vi "calibration.vi"(0 "信号时长[s]":dbl, 1 "Buffer":T1={"# buffers"=4, "Buffer size"=2048, "unit (ms)"=enum."Samples"}, 5 "终止频率[Hz]":dbl, 9 "起始频率[Hz]":dbl, 11 "信号幅值[V]":dbl, 13 "format":cluster{"Rate":i32, "Bits":i32, "Channels":u32}) -> ()   [LabVIEW 2021]
uses:
  Global.vi
  <vilib>/addons/_NISVFA/_Generation/SoundVib_Generation.lvlib
  <vilib>/Analysis/NI_AALPro.lvlib
  <vilib>/measure/NI_MABase.lvlib
panel:
  in  "Close Square":bool
  in  "校准电压值":dbl[](array[numeric])
  in  "amp":dbl
  in  "开始校准":bool
  in  "Stop":bool
  in  "验证校准值":bool
  out "Calibration Curve":cluster{"X":dbl, "Y":dbl}[](graph)
  out "intercept":dbl
  out "slope":dbl
  out "校准中":string
  # "-step1:  将万用表调整到交流电压测试模式，将信号输出连接万用表；\n-step2：点击开始校准按钮，待万用表示数稳定，点击暂停按钮，记录最大测量电压值；\n-step3：将校准电压值填入弹出的对话框；\n-step4：重复step2-step3 3次，校准结束后软件自动计算校准曲线；\n-step5：点击验证校准值，查看万用表示数是否与信号幅值相同；\n-step6：点击暂停并选择是否保存校准曲线"
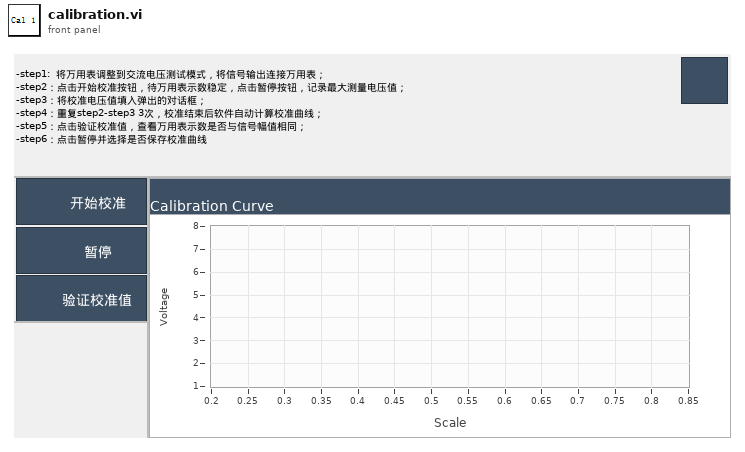
[diagram p1: front panel]
types:
  T1 = cluster{"# buffers":i32, "Buffer size":i32, "unit (ms)":enum16{"time (ms)", "Samples"}}
  T2 = cluster{"slope":dbl, "intercept":dbl, "校准电压值":dbl[]}
  T3 = typedef "SoundHandle.ctl" = cluster{"DeviceID":u16, "Samples/buf":u32, "Sampl rate":u32, "Bits/sample":u16, "Channels":u8, "Opened":bool}
  T4 = cluster{"start frequency [Hz]":dbl, "stop frequency [Hz]":dbl}
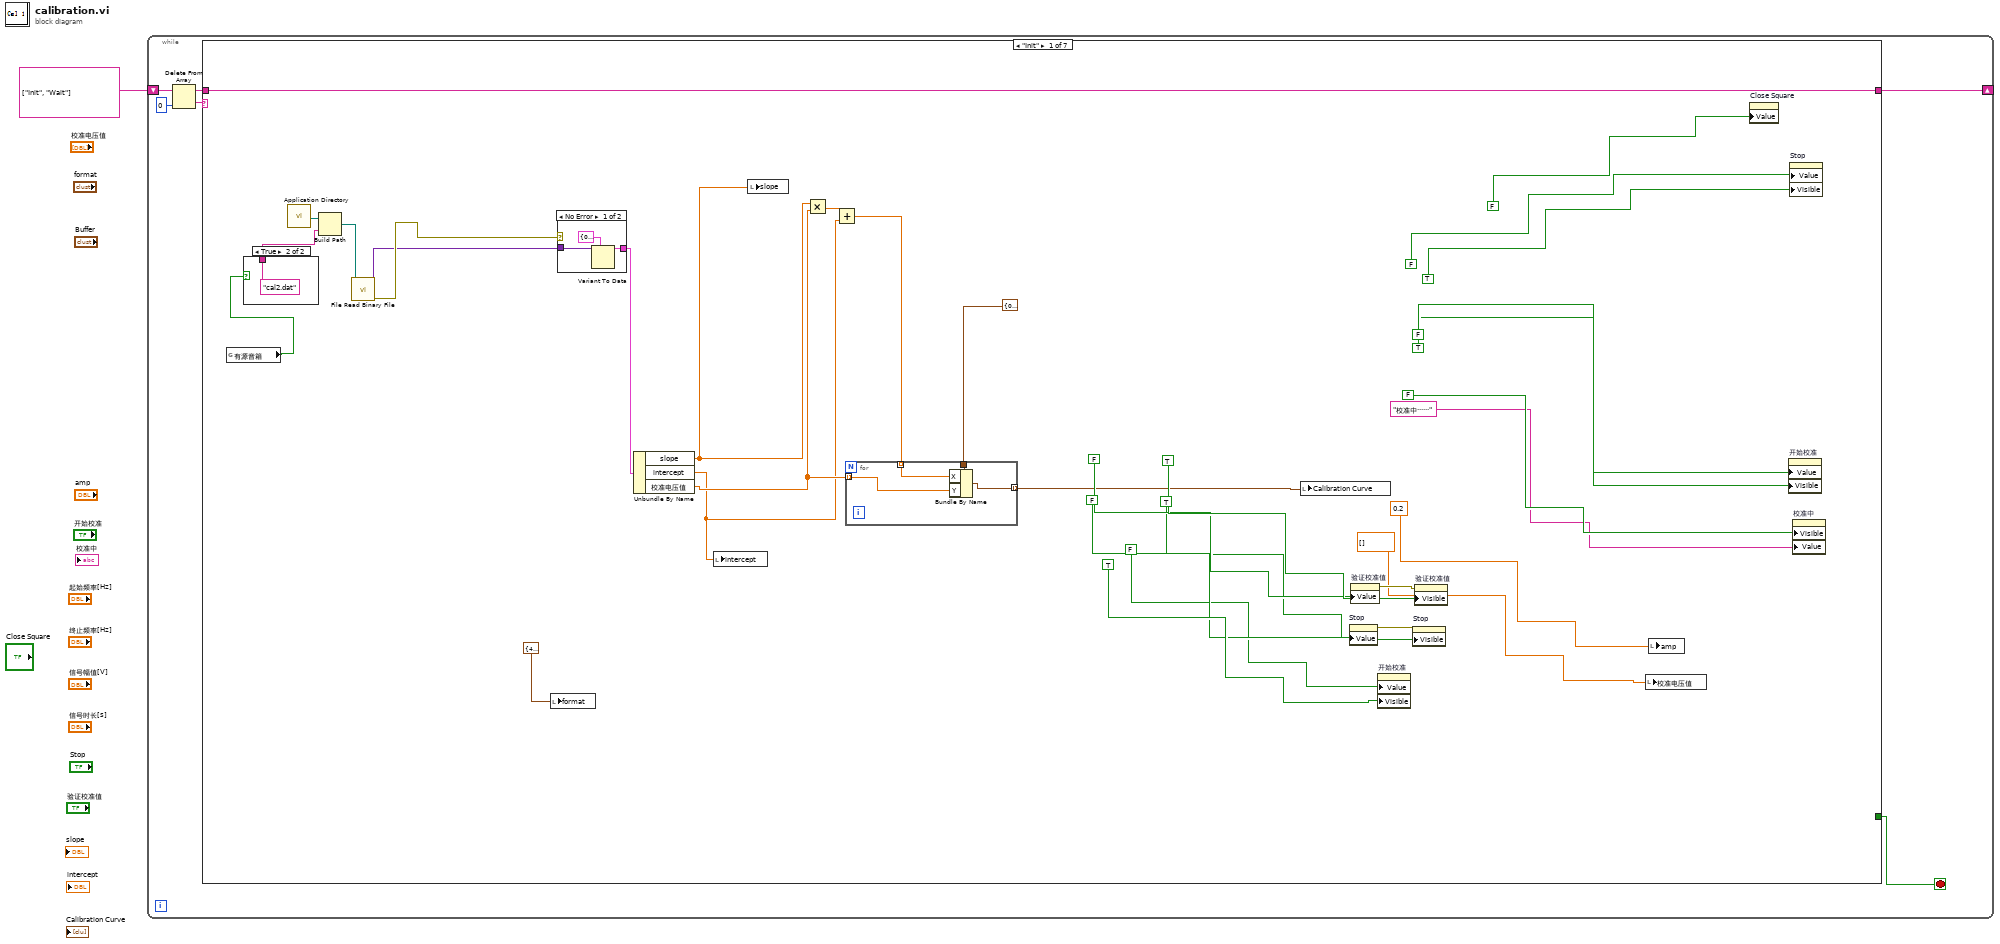
[diagram p0: block diagram]
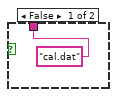
[diagram p2: hidden frame]
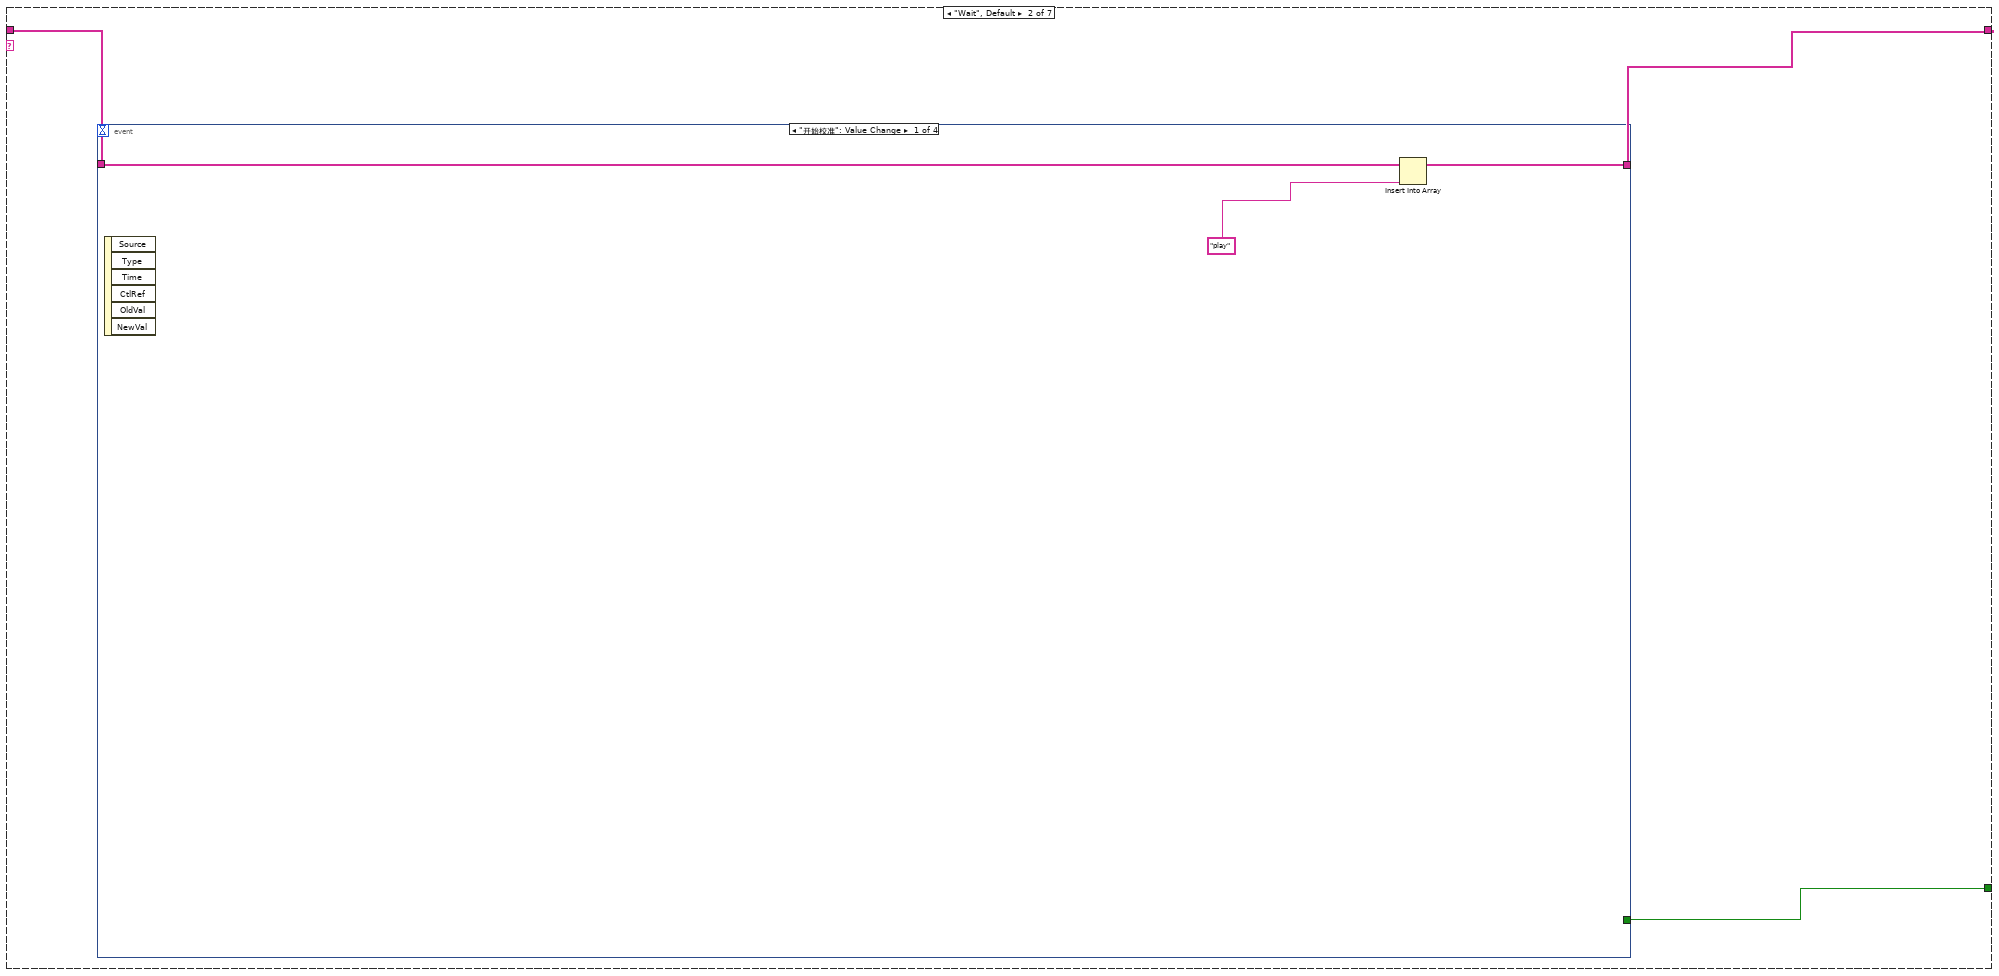
[diagram p4: hidden frame]
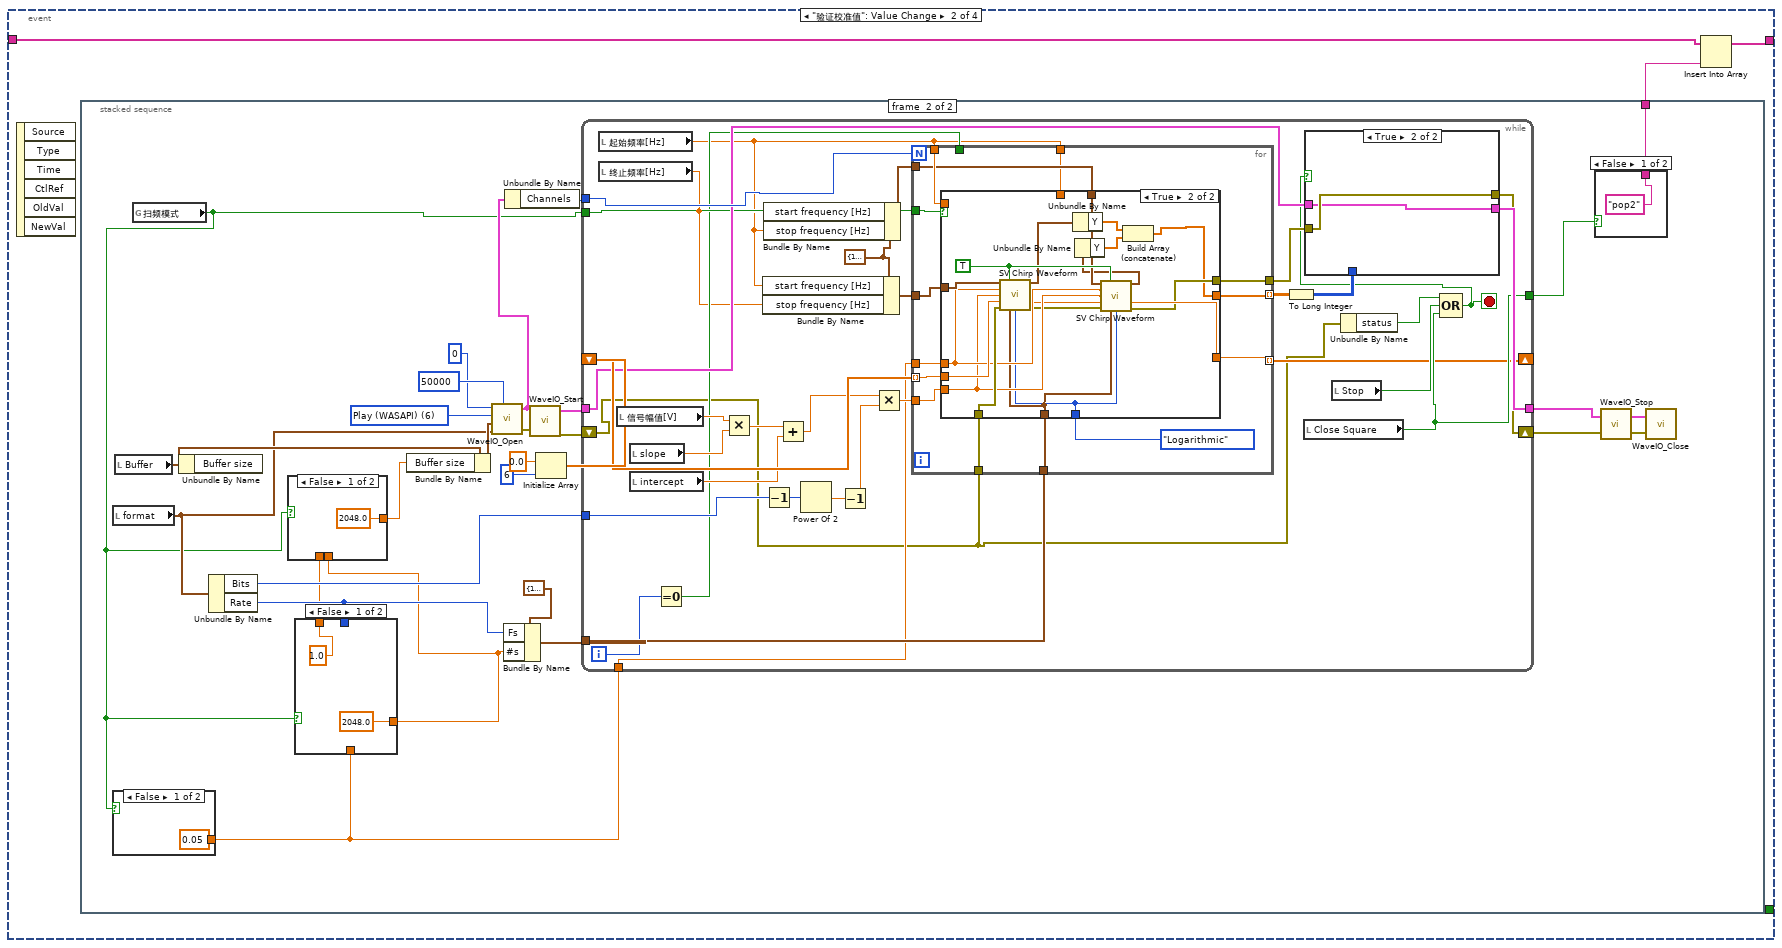
[diagram p5: hidden frame]
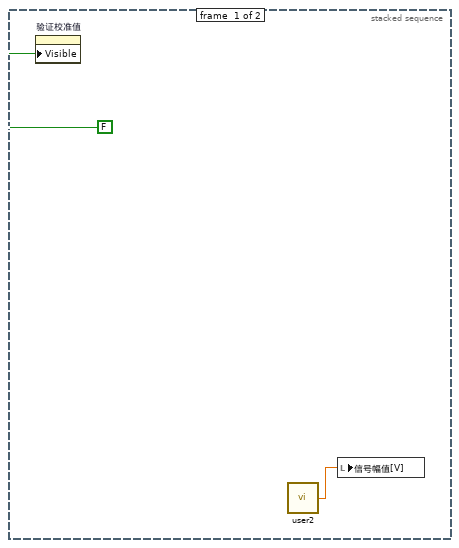
[diagram p6: hidden frame]
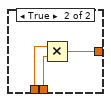
[diagram p7: hidden frame]
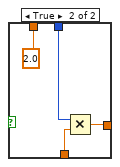
[diagram p8: hidden frame]
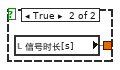
[diagram p9: hidden frame]
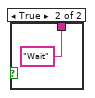
[diagram p10: hidden frame]
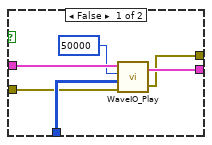
[diagram p11: hidden frame]
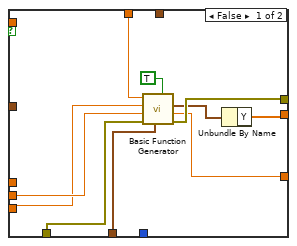
[diagram p12: hidden frame]
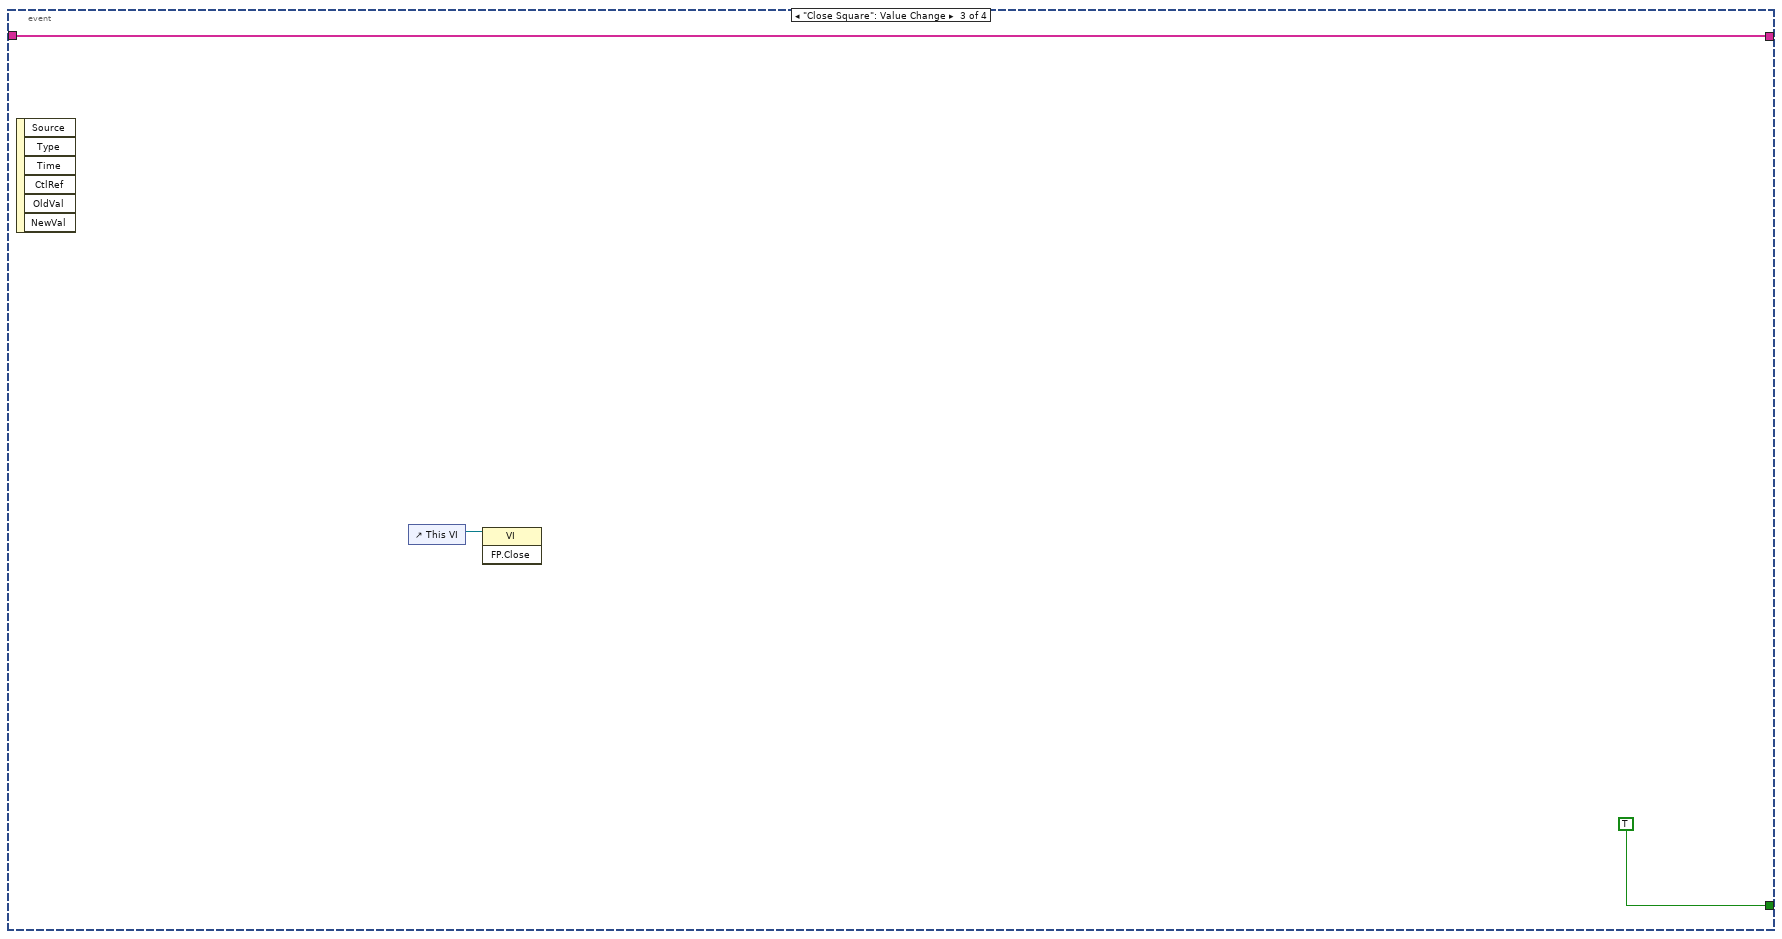
[diagram p13: hidden frame]
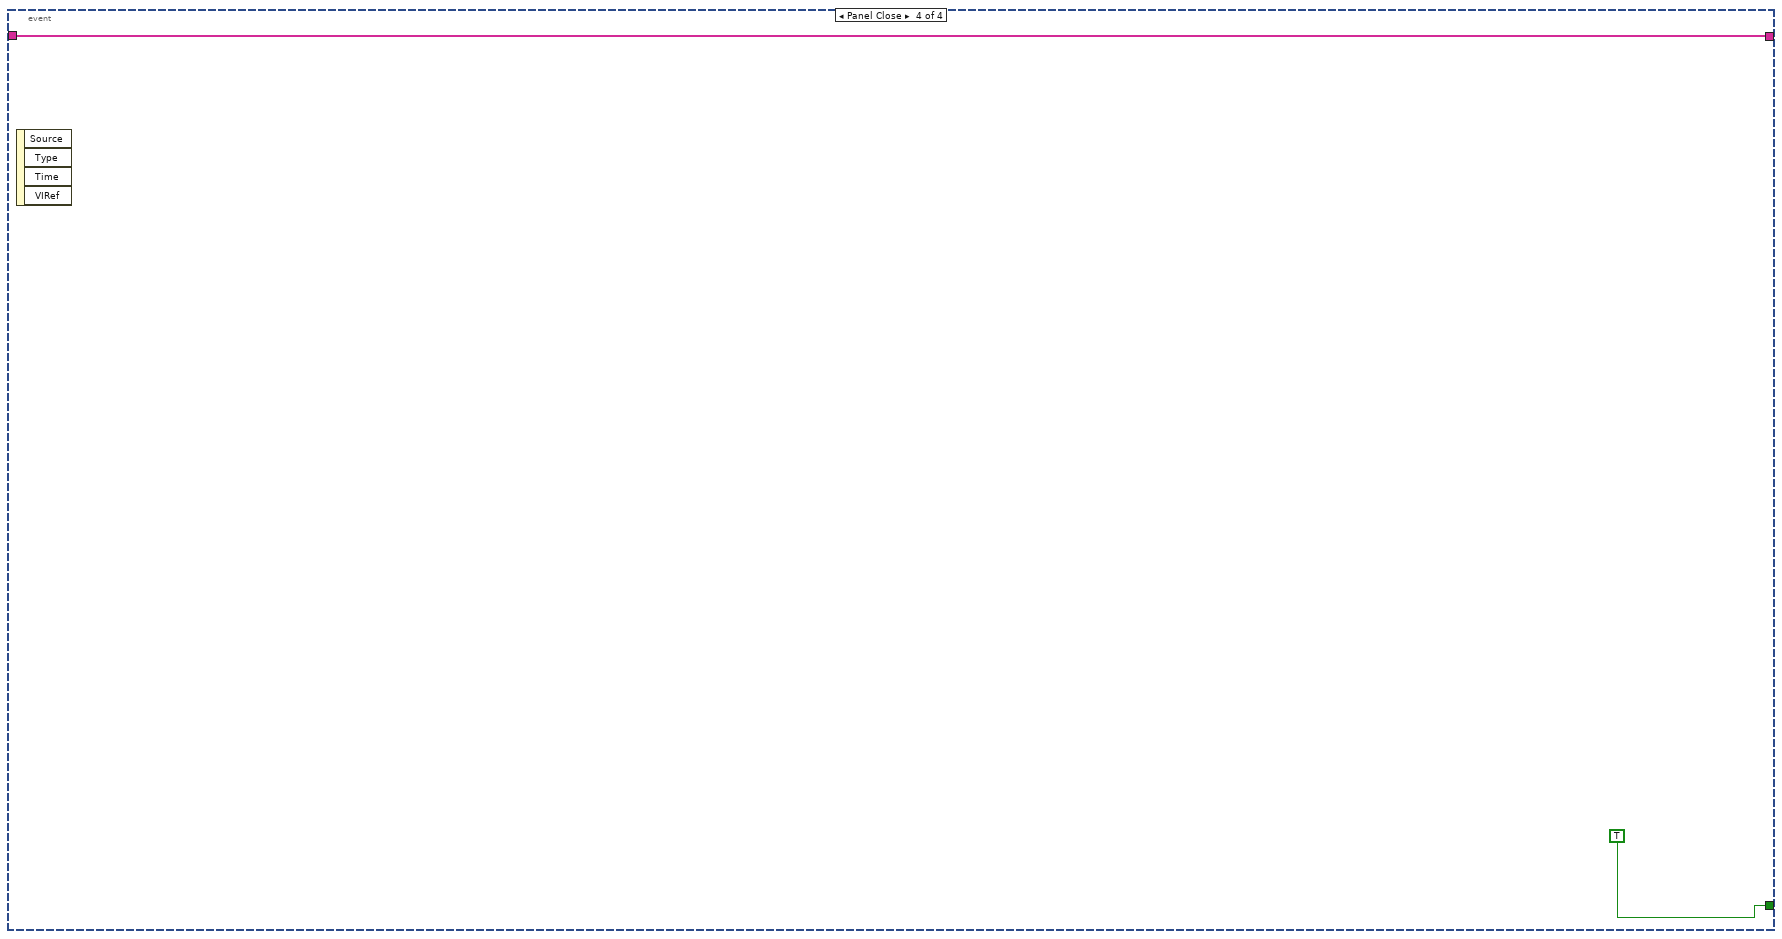
[diagram p14: hidden frame]
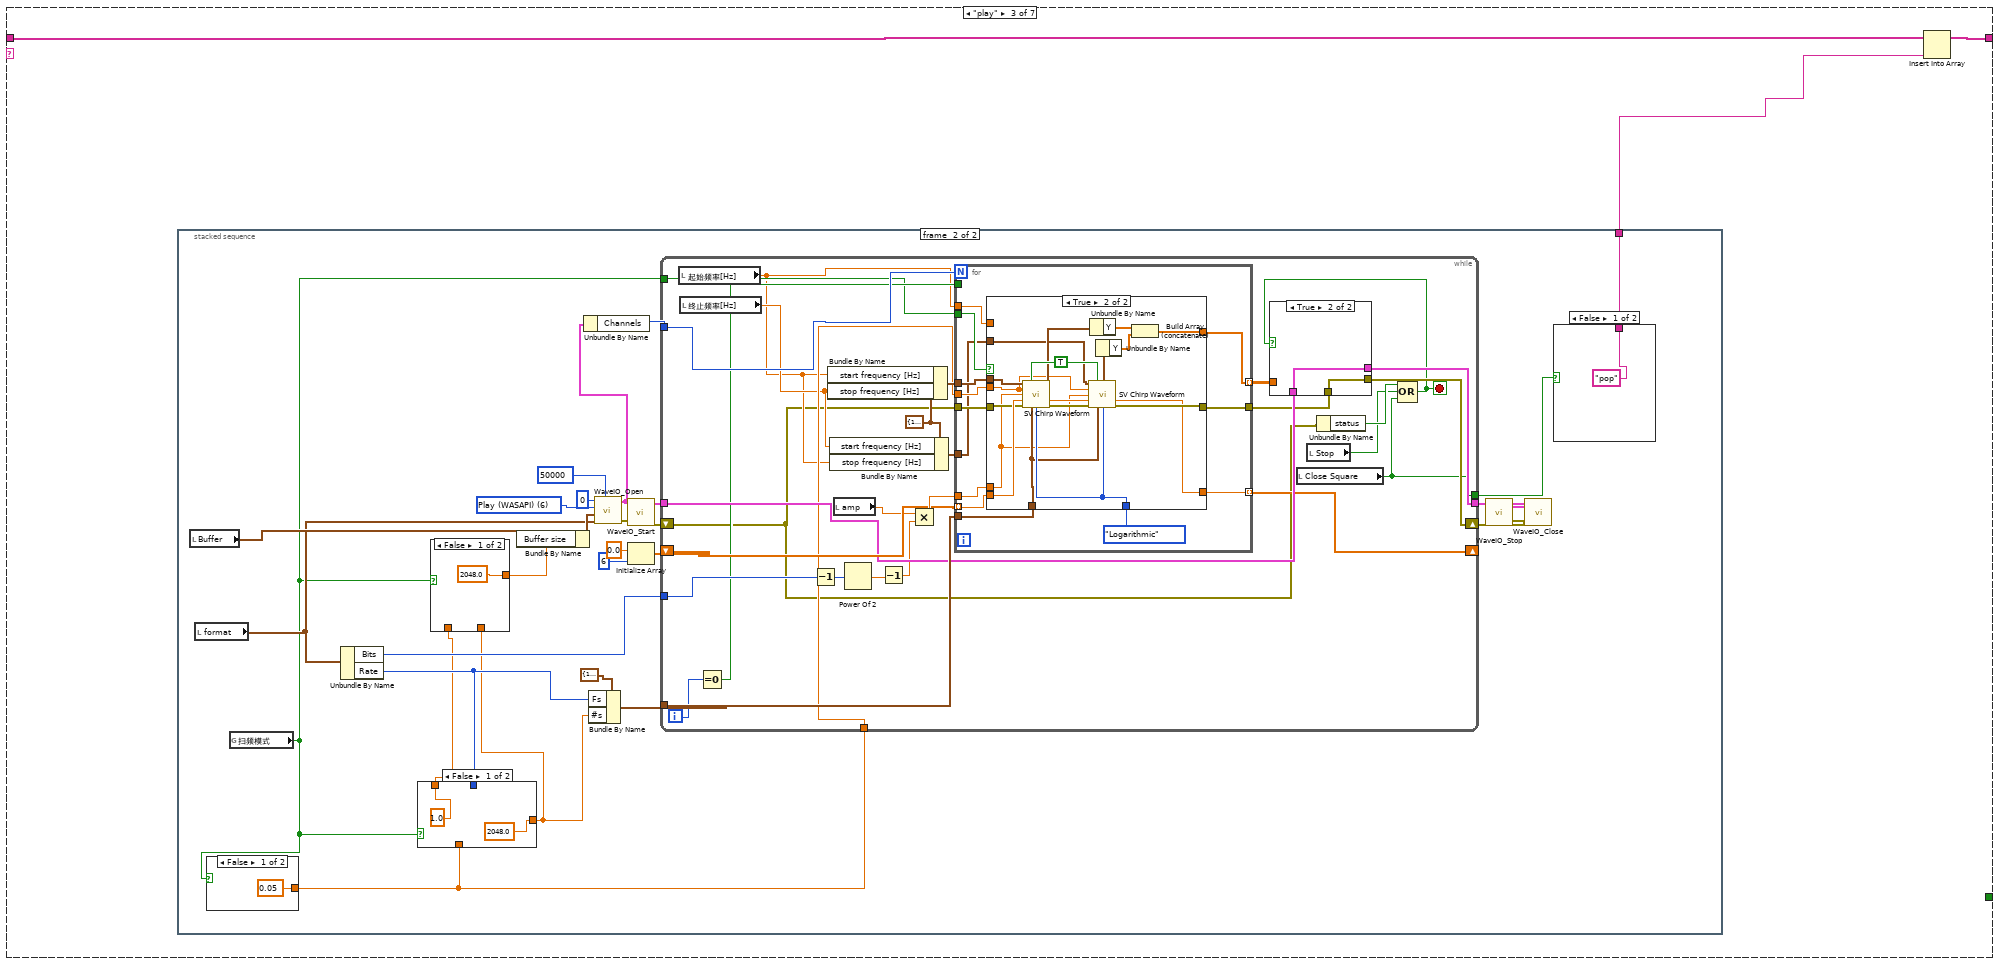
[diagram p15: hidden frame]
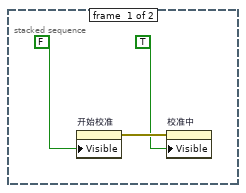
[diagram p16: hidden frame]
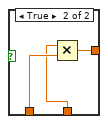
[diagram p17: hidden frame]
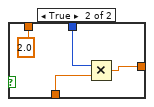
[diagram p18: hidden frame]
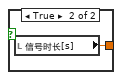
[diagram p19: hidden frame]
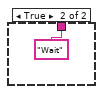
[diagram p20: hidden frame]
diagram:
  n1 = while {
    shift-right: [w3] -> _
    shift-left: string[] ["Init", "Wait"] -> [w6]
    stop <- w2 stop-if-true
    n2 = Delete From Array(array=w6, index=0 ("索引")) -> (deleted portion=w5:string, array with subset deleted=w4:string[])  [unwired: 1 in]
    n3 = case shown="\"Init\"" w5 {
      tunnel: [_ w50 _ TRUE _ _ _] -> w2
      tunnel: w4 -> [w31 w52 w195 w320 w328 w345 w386]
      tunnel: [w31 w51 w194 w320 w326 w344 w386] -> w3
      frame "Init" {
        n4 = global read "Global.vi" "有源音箱"() -> (w8:bool)
        n5 = case shown="True" w8 {
          tunnel: ["cal.dat" ("名称或相对路径") "cal2.dat" ("名称或相对路径")] -> w23
          frame False {
          }
          frame True {
          }
        }
        n6 = call <vilib>:"Application Directory.vi"() -> ("Application Directory"=w24:path)
        n7 = Build Path(base path=w24, name or relative path=w23) -> (appended path=w25:path)
        n8 = call "File Read Binary File.vi"("file path"=w25) -> ("error Output"=w28:errorcluster, "Variant Output"=w26:variant)  [unwired: 8 in, 1 out]
        n9 = local write "format"(cluster{"Rate":i32, "Bits":i32, "Channels":u32} {"Rate"=44100, "Bits"=24, "Channels"=2} ("format")) -> ()
        n10 = case shown="No Error" w28 {
          tunnel: w26 -> [w49 _]
          tunnel: [w48 _] -> w27
          frame No Error {
            n11 = Variant To Data(type=T2 {"slope"=0.0, "intercept"=0.0, "校准电压值"=[3.37, 6.73, 10.1, 13.48]}, Variant=w49) -> (data=w48:T2)  [unwired: 1 in, 1 out]
          }
          frame Error {
          }
        }
        n12 = Unbundle By Name(w27) -> ("slope"=w17:dbl, "intercept"=w16:dbl, "校准电压值"=w18:dbl[])
        n13 = local write "intercept"(w16) -> ()
        n14 = local write "slope"(w17) -> ()
        n15 = Multiply(x=w17, y=w18) -> (x*y=w22:dbl[])
        n16 = Add(x=w22, y=w16) -> (x+y=w21:dbl[])
        n17 = for {
          tunnel: cluster{"X":dbl, "Y":dbl} {"X"=0.0, "Y"=0.0} -> [w46]
          tunnel: w18 -> [w43] mode=indexing
          tunnel: w21 -> [w44] mode=indexing
          tunnel: [w45] -> w20 mode=indexing
          n18 = Bundle By Name(cluster=w46, "X"=w44, "Y"=w43) -> (w45:cluster{"X":dbl, "Y":dbl})
        }
        n19 = local write "Calibration Curve"(w20) -> ()
        n20 = property on="Stop" class="Bool (strict)"("Value"=FALSE ("可见")) -> (error out=w11:errorcluster)  [unwired: 2 in, 1 out]
        n21 = property on="验证校准值" class="Bool (strict)"("Value"=FALSE ("可见")) -> (error out=w40:errorcluster)  [unwired: 2 in, 1 out]
        n22 = property on="开始校准" class="Bool (strict)"("Value"=FALSE ("开始校准"), "Visible"=TRUE) -> ()  [unwired: 2 in, 2 out]
        n23 = property on="Stop" class="Bool (strict)"(error in=w11, "Visible"=TRUE) -> ()  [unwired: 1 in, 2 out]
        n24 = property on="验证校准值" class="Bool (strict)"(error in=w40, "Visible"=TRUE) -> ()  [unwired: 1 in, 2 out]
        n25 = local write "校准电压值"(dbl[] [] ("Array")) -> ()
        n26 = local write "amp"(0.2 ("amp")) -> ()
        n27 = property on="Close Square" class="Bool (strict)"("Value"=FALSE ("Close Square")) -> ()  [unwired: 2 in, 2 out]
        n28 = property on="开始校准" class="Bool (strict)"("Value"=FALSE, "Visible"=TRUE ("可见")) -> ()  [unwired: 2 in, 2 out]
        n29 = property on="Stop" class="Bool (strict)"("Value"=FALSE ("Stop"), "Visible"=TRUE) -> ()  [unwired: 2 in, 2 out]
        n30 = property on="校准中" class="Str"("Visible"=FALSE ("可见"), "Value"="校准中······" ("校准中")) -> ()  [unwired: 2 in, 2 out]
      }
      frame "Wait", Default {
        n31 = event shown="[0] \"开始校准\": Value Change" {
          selector: _ -> [_ _ _ _]
          dyn-events: _ -> [_ _ _ _]
          timeout: _ -> [_ _ _ _]
          tunnel: [_ _ TRUE TRUE] -> w50
          tunnel: [w54 w56 w188 w191] -> w51
          tunnel: w52 -> [w55 w58 w188 w191]
          event "开始校准": Value Change {
            n32 = event-data() -> ()  [unwired: 1 in, 6 out]
            n33 = Insert Into Array(array=w55, new element="play" ("new element/subarray")) -> (w54:string[])  [unwired: 1 in]
          }
          event "验证校准值": Value Change {
            n34 = event-data() -> ()  [unwired: 1 in, 6 out]
            n35 = stacked-sequence {
              tunnel: [_ w66] -> w57
              frame #0 {
                n36 = property on="验证校准值" class="Bool (strict)"("Visible"=FALSE ("可见")) -> ()  [unwired: 2 in, 2 out]
                n37 = call "user2.vi"() -> ("Numeric"=w59:dbl)
                n38 = local write "信号幅值[V]"(w59) -> ()
              }
              frame #1 {
                w72 = u16 6 items=["Record", "Play", "Loopback", "ASIO input", "ASIO output", "Record (WASAPI)", "Play (WASAPI)", "Record Combi", "Play Combi"] ("device type (Record)")
                n39 = local read "format"() -> (w68:cluster{"Rate":i32, "Bits":i32, "Channels":u32})
                n40 = local read "Buffer"() -> (w69:T1)
                n41 = global read "Global.vi" "扫频模式"() -> (w61:bool)
                n42 = case shown="False" w61 {
                  tunnel: [0.05 ("信号时长[s]") w101] -> w64
                  frame False {
                  }
                  frame True {
                    n43 = local read "信号时长[s]"() -> (w101:dbl)
                  }
                }
                n44 = Unbundle By Name(w69) -> ()  [unwired: 1 out]
                n45 = Unbundle By Name(w68) -> ("Bits"=w80:i32, "Rate"=w65:i32)
                n46 = case shown="False" w61 {
                  tunnel: [2048.0 w99] -> w63
                  tunnel: w65 -> [_ w98]
                  tunnel: w64 -> [_ w97]
                  tunnel: [1.0 ("x") 2.0 ("x")] -> w62
                  frame False {
                  }
                  frame True {
                    n47 = Multiply(x=w98, y=w97) -> (x*y=w99:dbl)
                  }
                }
                n48 = case shown="False" w61 {
                  tunnel: [2048.0 w93] -> w70
                  tunnel: w63 -> [_ w92]
                  tunnel: w62 -> [_ w91]
                  frame False {
                  }
                  frame True {
                    n49 = Multiply(x=w91, y=w92) -> (x*y=w93:dbl)
                  }
                }
                n50 = Bundle By Name(cluster=w69, "Buffer size"=w70) -> (w71:T1)
                n51 = call "WaveIO_Open.vi"("idev"=u32 0, "Watchdog timeout (msec) (default=OFF)"=50000, "device type (Record)"=w72, "Buffer Config"=w71, "Format (44kHz, 16Bit, stereo)"=w68) -> ("Sound Handle Out"=w75:T3, "error out"=w82:errorcluster)  [unwired: 2 in]
                n52 = Bundle By Name(cluster=cluster{"Fs":dbl, "#s":dbl} {"Fs"=1000.0, "#s"=1000.0} ("sampling info"), "Fs"=w65, "#s"=w63) -> (w85:cluster{"Fs":dbl, "#s":dbl})
                n53 = Unbundle By Name(w75) -> ("Channels"=w74:u8)
                n54 = call "WaveIO_Start.vi"("error in (no error)"=w82, "Handle"=w75) -> ("error out"=w83:errorcluster, "Handle Out"=w84:T3)
                n55 = Initialize Array(0.0 ("element"), 6 ("dimension size")) -> (w79:dbl[])
                n56 = while {
                  shift-right: [w129] -> w81
                  shift-left: w83 -> [w105]
                  tunnel: w84 -> [w127]
                  tunnel: [w136] -> w88
                  tunnel: w85 -> [w137]
                  tunnel: w80 -> [w135]
                  shift-right: [w107] -> _
                  shift-left: w79 -> [w130]
                  tunnel: w74 -> [w128]
                  tunnel: w64 -> [w123]
                  tunnel: [w115] -> w67
                  tunnel: w61 -> [w113]
                  i -> [w112]
                  stop <- w104 stop-if-true
                  w110 = T4 {"start frequency [Hz]"=10.0, "stop frequency [Hz]"=10000.0} ("frequency range")
                  n57 = local read "起始频率[Hz]"() -> (w106:dbl)
                  n58 = local read "终止频率[Hz]"() -> (w109:dbl)
                  n59 = local read "信号幅值[V]"() -> (w122:dbl)
                  n60 = local read "slope"() -> (w121:dbl)
                  n61 = local read "intercept"() -> (w119:dbl)
                  n62 = Equal To 0?(x=w112) -> (x = 0?=w111:bool)
                  n63 = Multiply(x=w122, y=w121) -> (x*y=w120:dbl)
                  n64 = Bundle By Name(cluster=w110, "start frequency [Hz]"=w106, "stop frequency [Hz]"=w109) -> (w124:T4)
                  n65 = Bundle By Name(cluster=w110, "start frequency [Hz]"=w109, "stop frequency [Hz]"=w106) -> (w108:T4)
                  n66 = Decrement(x=w135) -> (x-1=w134:i32)
                  n67 = Add(x=w120, y=w119) -> (x+y=w118:dbl)
                  n68 = Power Of 2(x=w134) -> (2^x=w117:dbl)
                  n69 = Decrement(x=w117) -> (x-1=w116:dbl)
                  n70 = Multiply(x=w118, y=w116) -> (x*y=w133:dbl)
                  n71 = for {
                    N: w128 -> [_]
                    tunnel: w137 -> [w158]
                    tunnel: w133 -> [w157]
                    tunnel: [w147] -> w132 mode=indexing
                    tunnel: w130 -> [w159] mode=indexing
                    tunnel: w124 -> [w156]
                    tunnel: w123 -> [w155]
                    tunnel: w105 -> [w153]
                    tunnel: [w152] -> w114
                    tunnel: w106 -> [w151]
                    tunnel: w113 -> [w150]
                    tunnel: w111 -> [_]
                    tunnel: w108 -> [w149]
                    tunnel: [w148] -> w107 mode=indexing
                    tunnel: w106 -> [w146]
                    n72 = case shown="True" w150 {
                      tunnel: w159 -> [w167 w187]
                      tunnel: w158 -> [w168 w171]
                      tunnel: [w162 w170] -> w147
                      tunnel: w157 -> [w166 w181]
                      tunnel: w156 -> [_ w186]
                      tunnel: w155 -> [_ w182]
                      tunnel: enum16{"Linear", "Logarithmic"}."Logarithmic" ("frequency spacing") -> [_ w172]
                      tunnel: w151 -> [_ _]
                      tunnel: w153 -> [w160 w185]
                      tunnel: [w169 w173] -> w152
                      tunnel: w149 -> [_ w183]
                      tunnel: [w161 w179] -> w148
                      tunnel: w146 -> [w165 _]
                      frame False {
                        n73 = call <vilib>:"Basic Function Generator.vi"("reset signal"=TRUE, "sampling info"=w168, "error in (no error)"=w160, "phase"=w167, "amplitude"=w166, "frequency"=w165) -> ("error out"=w169:errorcluster, "phase out"=w161:dbl, "signal out"=w163:waveform(dbl))  [unwired: 3 in]
                        n74 = Unbundle By Name(w163) -> ("Y"=w162:dbl[])
                      }
                      frame True {
                        w184 = TRUE ("reset signal (F)")
                        n75 = call <vilib>:"SV Chirp Waveform.vi"("frequency range"=w186, "reset signal (F)"=w184, "chirp duration [s]"=w182, "amplitude"=w181, "phase in [deg]"=w187, "error in (no error)"=w185, "sampling info"=w171, "frequency spacing"=w172) -> ("chirp signal"=w175:waveform(dbl), "phase out [deg]"=w180:dbl, "error out"=w174:errorcluster)  [unwired: 5 in]
                        n76 = Unbundle By Name(w175) -> ("Y"=w177:dbl[])
                        n77 = call <vilib>:"SV Chirp Waveform.vi"("frequency range"=w183, "reset signal (F)"=w184, "chirp duration [s]"=w182, "amplitude"=w181, "phase in [deg]"=w180, "error in (no error)"=w174, "sampling info"=w171, "frequency spacing"=w172) -> ("chirp signal"=w178:waveform(dbl), "phase out [deg]"=w179:dbl, "error out"=w173:errorcluster)  [unwired: 5 in]
                        n78 = Unbundle By Name(w178) -> ("Y"=w176:dbl[])
                        n79 = Build Array (concatenate)(w177, w176) -> (w170:dbl[])
                      }
                    }
                  }
                  n80 = To Long Integer(number=w132) -> (32bit integer=w131:i32[][])
                  n81 = local read "Close Square"() -> (w115:bool)
                  n82 = local read "Stop"() -> (w125:bool)
                  n83 = Unbundle By Name(w105) -> ("status"=w126:bool)
                  n84 = Compound Arithmetic op=OR(w126, w125, w115) -> (w104:bool)
                  n85 = case shown="True" w104 {
                    tunnel: [w143 w144] -> w136
                    tunnel: w131 -> [w142 _]
                    tunnel: [w141 w145] -> w129
                    tunnel: w127 -> [w140 w144]
                    tunnel: w114 -> [w139 w145]
                    frame False {
                      n86 = call "WaveIO_Play.vi"("error in (no error)"=w139, "data"=w142, "timeout (automatic)"=50000, "Handle"=w140) -> ("error out"=w141:errorcluster, "Handle Out"=w143:T3)
                    }
                    frame True {
                    }
                  }
                }
                n87 = case shown="False" w67 {
                  tunnel: ["pop2" "Wait"] -> w66
                  frame False {
                  }
                  frame True {
                  }
                }
                n88 = call "WaveIO_Stop.vi"("error in (no error)"=w81, "Handle"=w88) -> ("error out"=w87:errorcluster, "Handle Out"=w89:T3)
                n89 = call "WaveIO_Close.vi"("error in (no error)"=w87, "Handle"=w89) -> ()  [unwired: 2 out]
              }
            }
            n90 = Insert Into Array(array=w58, new element=w57) -> (w56:string[])  [unwired: 1 in]
          }
          event "Close Square": Value Change {
            n91 = event-data() -> ()  [unwired: 1 in, 6 out]
            n92 = control-ref of="This VI"() -> (w189:refnum<vi>)
            n93 = invoke class="VI" method="FP.Close"(reference=w189) -> ()  [unwired: 2 in, 3 out]
          }
          event Panel Close {
            n94 = event-data() -> ()  [unwired: 1 in, 4 out]
          }
        }
      }
      frame "play" {
        n95 = stacked-sequence {
          tunnel: [_ w227] -> w193
          frame #0 {
            n96 = property on="开始校准" class="Bool (strict)"("Visible"=FALSE ("可见")) -> (error out=w198:errorcluster)  [unwired: 2 in, 1 out]
            n97 = property on="校准中" class="Str"(error in=w198, "Visible"=TRUE) -> ()  [unwired: 1 in, 2 out]
          }
          frame #1 {
            w209 = u16 6 items=["Record", "Play", "Loopback", "ASIO input", "ASIO output", "Record (WASAPI)", "Play (WASAPI)", "Record Combi", "Play Combi"] ("device type (Record)")
            n98 = local read "Buffer"() -> (w207:T1)
            n99 = local read "format"() -> (w206:cluster{"Rate":i32, "Bits":i32, "Channels":u32})
            n100 = global read "Global.vi" "扫频模式"() -> (w199:bool)
            n101 = case shown="False" w199 {
              tunnel: [0.05 ("信号时长[s]") w239] -> w203
              frame False {
              }
              frame True {
                n102 = local read "信号时长[s]"() -> (w239:dbl)
              }
            }
            n103 = Unbundle By Name(w206) -> ("Bits"=w217:i32, "Rate"=w202:i32)
            n104 = case shown="False" w199 {
              tunnel: [2048.0 w237] -> w200
              tunnel: w203 -> [_ w236]
              tunnel: w202 -> [_ w235]
              tunnel: [1.0 2.0] -> w201
              frame False {
              }
              frame True {
                n105 = Multiply(x=w235, y=w236) -> (x*y=w237:dbl)
              }
            }
            n106 = case shown="False" w199 {
              tunnel: [2048.0 w231] -> w204
              tunnel: w201 -> [_ w230]
              tunnel: w200 -> [_ w229]
              frame False {
              }
              frame True {
                n107 = Multiply(x=w229, y=w230) -> (x*y=w231:dbl)
              }
            }
            n108 = Bundle By Name(cluster=w207, "Buffer size"=w204) -> (w208:T1)
            n109 = Bundle By Name(cluster=cluster{"Fs":dbl, "#s":dbl} {"Fs"=1000.0, "#s"=1000.0} ("sampling info"), "Fs"=w202, "#s"=w200) -> (w222:cluster{"Fs":dbl, "#s":dbl})
            n110 = call "WaveIO_Open.vi"("idev"=u32 0, "Watchdog timeout (msec) (default=OFF)"=50000, "device type (Record)"=w209, "Buffer Config"=w208, "Format (44kHz, 16Bit, stereo)"=w206) -> ("Sound Handle Out"=w212:T3, "error out"=w219:errorcluster)  [unwired: 2 in]
            n111 = Unbundle By Name(w212) -> ("Channels"=w211:u8)
            n112 = call "WaveIO_Start.vi"("error in (no error)"=w219, "Handle"=w212) -> ("error out"=w220:errorcluster, "Handle Out"=w221:T3)
            n113 = Initialize Array(0.0 ("element"), 6 ("dimension size")) -> (w216:dbl[])
            n114 = while {
              shift-right: [w264] -> w218
              shift-left: w220 -> [w243]
              tunnel: w221 -> [w262]
              tunnel: [w269] -> w225
              tunnel: w222 -> [w270]
              tunnel: w217 -> [w268]
              shift-right: [w261] -> _
              shift-left: w216 -> [w265]
              tunnel: w211 -> [w263]
              tunnel: w203 -> [w258]
              tunnel: [w252] -> w205
              tunnel: w199 -> [w249]
              i -> [w251]
              stop <- w242 stop-if-true
              w247 = T4 {"start frequency [Hz]"=10.0, "stop frequency [Hz]"=10000.0} ("frequency range")
              n115 = local read "起始频率[Hz]"() -> (w245:dbl)
              n116 = local read "终止频率[Hz]"() -> (w246:dbl)
              n117 = Equal To 0?(x=w251) -> (x = 0?=w250:bool)
              n118 = Decrement(x=w268) -> (x-1=w267:i32)
              n119 = Bundle By Name(cluster=w247, "start frequency [Hz]"=w245, "stop frequency [Hz]"=w246) -> (w259:T4)
              n120 = Bundle By Name(cluster=w247, "start frequency [Hz]"=w246, "stop frequency [Hz]"=w245) -> (w244:T4)
              n121 = local read "amp"() -> (w256:dbl)
              n122 = Power Of 2(x=w267) -> (2^x=w257:dbl)
              n123 = Decrement(x=w257) -> (x-1=w254:dbl)
              n124 = Multiply(x=w256, y=w254) -> (x*y=w266:dbl)
              n125 = for {
                N: w263 -> [_]
                tunnel: w270 -> [w290]
                tunnel: w266 -> [w289]
                tunnel: [w281] -> w255 mode=indexing
                tunnel: w265 -> [w292] mode=indexing
                tunnel: [w291] -> w261 mode=indexing
                tunnel: w259 -> [w288]
                tunnel: w258 -> [w287]
                tunnel: w250 -> [_]
                tunnel: w249 -> [w285]
                tunnel: w245 -> [w284]
                tunnel: w243 -> [w283]
                tunnel: [w282] -> w248
                tunnel: w244 -> [w280]
                n126 = case shown="True" w285 {
                  tunnel: w292 -> [w299 w319]
                  tunnel: [w295 w314] -> w291
                  tunnel: w290 -> [w296 w312]
                  tunnel: w289 -> [w300 w306]
                  tunnel: w288 -> [_ w318]
                  tunnel: w287 -> [_ w305]
                  tunnel: enum16{"Linear", "Logarithmic"}."Logarithmic" ("frequency spacing") -> [_ w313]
                  tunnel: w284 -> [w301 _]
                  tunnel: w283 -> [w298 w316]
                  tunnel: [w297 w317] -> w282
                  tunnel: [w294 w303] -> w281
                  tunnel: w280 -> [_ w304]
                  frame False {
                    n127 = call <vilib>:"Basic Function Generator.vi"("reset signal"=TRUE, "sampling info"=w296, "error in (no error)"=w298, "phase"=w299, "amplitude"=w300, "frequency"=w301) -> ("error out"=w297:errorcluster, "phase out"=w295:dbl, "signal out"=w293:waveform(dbl))  [unwired: 3 in]
                    n128 = Unbundle By Name(w293) -> ("Y"=w294:dbl[])
                  }
                  frame True {
                    w311 = TRUE ("reset signal (F)")
                    n129 = call <vilib>:"SV Chirp Waveform.vi"("frequency range"=w318, "reset signal (F)"=w311, "chirp duration [s]"=w305, "amplitude"=w306, "phase in [deg]"=w319, "error in (no error)"=w316, "sampling info"=w312, "frequency spacing"=w313) -> ("chirp signal"=w310:waveform(dbl), "phase out [deg]"=w315:dbl, "error out"=w317:errorcluster)  [unwired: 5 in]
                    n130 = call <vilib>:"SV Chirp Waveform.vi"("frequency range"=w304, "reset signal (F)"=w311, "chirp duration [s]"=w305, "amplitude"=w306, "phase in [deg]"=w315, "sampling info"=w312, "frequency spacing"=w313) -> ("chirp signal"=w309:waveform(dbl), "phase out [deg]"=w314:dbl)  [unwired: 6 in, 1 out]
                    n131 = Unbundle By Name(w310) -> ("Y"=w307:dbl[])
                    n132 = Unbundle By Name(w309) -> ("Y"=w308:dbl[])
                    n133 = Build Array (concatenate)(w307, w308) -> (w303:dbl[])
                  }
                }
              }
              n134 = local read "Close Square"() -> (w252:bool)
              n135 = local read "Stop"() -> (w253:bool)
              n136 = Unbundle By Name(w243) -> ("status"=w260:bool)
              n137 = Compound Arithmetic op=OR(w260, w253, w252) -> (w242:bool)
              n138 = case shown="True" w242 {
                tunnel: [w277 w279] -> w269
                tunnel: [w275 w278] -> w264
                tunnel: w262 -> [w274 w279]
                tunnel: w255 -> [w273 _]
                tunnel: w248 -> [w272 w278]
                frame False {
                  n139 = To Long Integer(number=w273) -> (32bit integer=w276:i32[][])
                  n140 = call "WaveIO_Play.vi"("error in (no error)"=w272, "data"=w276, "timeout (automatic)"=50000 ("Watchdog timeout (msec) (default=OFF)"), "Handle"=w274) -> ("error out"=w275:errorcluster, "Handle Out"=w277:T3)
                }
                frame True {
                }
              }
            }
            n141 = call "WaveIO_Stop.vi"("error in (no error)"=w218, "Handle"=w225) -> ("error out"=w224:errorcluster, "Handle Out"=w226:T3)
            n142 = call "WaveIO_Close.vi"("error in (no error)"=w224, "Handle"=w226) -> ()  [unwired: 2 out]
            n143 = case shown="False" w205 {
              tunnel: ["pop" "Wait"] -> w227
              frame False {
              }
              frame True {
              }
            }
          }
        }
        n144 = Insert Into Array(array=w195, new element=w193) -> (w194:string[])  [unwired: 1 in]
      }
      frame "Exit" {
        n145 = control-ref of="This VI"() -> (w322:refnum<vi>)
        n146 = invoke class="VI" method="FP.Close"(reference=w322) -> ()  [unwired: 2 in, 3 out]
      }
      frame "pop" {
        n147 = local read "校准电压值"() -> (w324:dbl[])
        n148 = call "user.vi"() -> ("Numeric"=w325:dbl)
        n149 = Insert Into Array(array=w324, new element=w325) -> (w323:dbl[])  [unwired: 1 in]
        n150 = local write "校准电压值"(w323) -> ()
        n151 = property on="开始校准" class="Bool (strict)"("Value"=FALSE, "Visible"=TRUE ("可见")) -> ()  [unwired: 2 in, 2 out]
        n152 = property on="校准中" class="Str"("Visible"=FALSE ("可见"), "Value"="校准中······" ("校准中")) -> ()  [unwired: 2 in, 2 out]
        n153 = property on="Stop" class="Bool (strict)"("Value"=FALSE ("Stop")) -> ()  [unwired: 2 in, 2 out]
        n154 = local read "amp"() -> (w335:dbl)
        n155 = Equal?(x=w335, y=0.8) -> (x = y?=w336:bool)
        n156 = case shown="False" w336 {
          tunnel: w335 -> [w340 _]
          tunnel: ["play" "Calculate"] -> w327
          frame False {
            n157 = Add(x=w340, y=0.2) -> (x+y=w338:dbl)
            n158 = local write "amp"(w338) -> ()
          }
          frame True {
            n159 = local write "amp"(0.2 ("amp")) -> ()
          }
        }
        n160 = Insert Into Array(array=w328, new element=w327) -> (w326:string[])  [unwired: 1 in]
      }
      frame "pop2" {
        n161 = Two Button Dialog(message="校准值是否准确", 1:"不准确，重新校准" ("F button name (\"Cancel\")"), 2:"准确，保存校准值" ("T button name (\"OK\")")) -> (T button?=w357:bool)
        n162 = case shown="True" w357 {
          frame False {
            n163 = local write "amp"(0.2 ("校准电压值[V] out")) -> ()
            n164 = local write "校准电压值"(dbl[] [] ("校准电压值")) -> ()
          }
          frame True {
            n165 = global read "Global.vi" "有源音箱"() -> (w361:bool)
            n166 = case shown="True" w361 {
              frame True {
                n167 = local read "校准电压值"() -> (w362:dbl[])
                n168 = local read "intercept"() -> (w363:dbl)
                n169 = local read "slope"() -> (w364:dbl)
                n170 = call <vilib>:"Application Directory.vi"() -> ("Application Directory"=w369:path)
                n171 = Bundle By Name(cluster=T2 {"slope"=0.0, "intercept"=0.0, "校准电压值"=[3.37, 6.73, 10.1, 13.48]}, "slope"=w364, "intercept"=w363, "校准电压值"=w362) -> (w365:T2)
                n172 = Build Path(base path=w369, name or relative path="cal2.dat") -> (appended path=w367:path)
                n173 = call "File Write to Variant.vi"("Input Data"=w365, "Path to Write"=w367) -> ()  [unwired: 5 in, 5 out]
              }
              frame False {
                n174 = local read "校准电压值"() -> (w370:dbl[])
                n175 = local read "intercept"() -> (w371:dbl)
                n176 = local read "slope"() -> (w372:dbl)
                n177 = call <vilib>:"Application Directory.vi"() -> ("Application Directory"=w377:path)
                n178 = Bundle By Name(cluster=T2 {"slope"=0.0, "intercept"=0.0, "校准电压值"=[3.37, 6.73, 10.1, 13.48]}, "slope"=w372, "intercept"=w371, "校准电压值"=w370) -> (w373:T2)
                n179 = Build Path(base path=w377, name or relative path="cal.dat") -> (appended path=w375:path)
                n180 = call "File Write to Variant.vi"("Input Data"=w373, "Path to Write"=w375) -> ()  [unwired: 5 in, 5 out]
              }
            }
          }
        }
        n181 = property on="验证校准值" class="Bool (strict)"("Value"=FALSE ("可见")) -> (error out=w358:errorcluster)  [unwired: 2 in, 1 out]
        n182 = property on="验证校准值" class="Bool (strict)"(error in=w358, "Visible"=TRUE) -> ()  [unwired: 1 in, 2 out]
        n183 = property on="开始校准" class="Bool (strict)"("Value"=FALSE, "Visible"=TRUE ("可见")) -> ()  [unwired: 2 in, 2 out]
        n184 = property on="Stop" class="Bool (strict)"("Value"=FALSE ("Stop"), "Visible"=TRUE) -> ()  [unwired: 2 in, 2 out]
        n185 = property on="校准中" class="Str"("Visible"=FALSE ("可见"), "Value"="校准中······" ("校准中")) -> ()  [unwired: 2 in, 2 out]
        n186 = Insert Into Array(array=w345, new element="Wait" ("new element/subarray")) -> (w344:string[])  [unwired: 1 in]
      }
      frame "Calculate" {
        n187 = local read "校准电压值"() -> (w380:dbl[])
        n188 = call <vilib>:"Linear Fit.vi"("Y"=dbl[] [0.2, 0.4, 0.6, 0.8], "X"=w380) -> ("slope"=w384:dbl, "intercept"=w382:dbl)  [unwired: 9 in, 3 out]
        n189 = Multiply(x=w384, y=w380) -> (x*y=w383:dbl[])
        n190 = local write "slope"(w384) -> ()
        n191 = local write "intercept"(w382) -> ()
        n192 = Add(x=w383, y=w382) -> (x+y=w379:dbl[])
        n193 = for {
          tunnel: cluster{"X":dbl, "Y":dbl} {"X"=0.0, "Y"=0.0} -> [w390]
          tunnel: w380 -> [w388] mode=indexing
          tunnel: w379 -> [w387] mode=indexing
          tunnel: [w389] -> w378 mode=indexing
          n194 = Bundle By Name(cluster=w390, "X"=w387, "Y"=w388) -> (w389:cluster{"X":dbl, "Y":dbl})
        }
        n195 = local write "Calibration Curve"(w378) -> ()
      }
    }
  }
